vi "AprilTag Desktop.vi"() -> ()   [LabVIEW 2025]
uses:
  <vilib>/Serenial/G Augmented-Reality Toolkit/g_ar_toolkit.feature_detection/Apriltag Detector/Detector Settings.ctl
  <vilib>/Serenial/G Augmented-Reality Toolkit/g_ar_toolkit.capture/Stream/Stream.lvclass/Stream.ctl
  <vilib>/Serenial/G Augmented-Reality Toolkit/g_ar_toolkit.image/New Image (ARGB Preallocated).vi
  <vilib>/Serenial/G Augmented-Reality Toolkit/g_ar_toolkit.image/New Image (Greyscale Preallocated).vi
  <vilib>/Serenial/G Augmented-Reality Toolkit/g_ar_toolkit.capture/Stream/Next Capture (ARGB).vi
  <vilib>/Serenial/G Augmented-Reality Toolkit/g_ar_toolkit.image/Draw Image to Picture (ARGB).vi
  <vilib>/Serenial/G Augmented-Reality Toolkit/g_ar_toolkit.image/ARGB Colour to U32 Pixel Value.vi
  <vilib>/Serenial/G Augmented-Reality Toolkit/g_ar_toolkit.common/NI-Linux-RT Shared Library Path (Core).vi
  <vilib>/Serenial/G Augmented-Reality Toolkit/g_ar_toolkit.image/ARGBExtractChannel.vi
  <vilib>/Serenial/G Augmented-Reality Toolkit/g_ar_toolkit.common/NI-Linux-RT Shared Library Path.vi
  <vilib>/Utility/error.llb/Error Cluster From Error Code.vi
  <vilib>/Serenial/G Augmented-Reality Toolkit/g_ar_toolkit.capture/Stream/Stream.lvclass
  <vilib>/Serenial/G Augmented-Reality Toolkit/g_ar_toolkit.capture/g_ar_toolkit.capture.lvlib
  <vilib>/Serenial/G Augmented-Reality Toolkit/g_ar_toolkit.image/g_ar_toolkit.image.lvlib
  <vilib>/ptbypt/NI_PtbyPt.lvlib
  <vilib>/Serenial/G Augmented-Reality Toolkit/g_ar_toolkit.feature_detection/Apriltag Detector/AprilTag Detector.lvclass
panel:
  out "error out 3":errorcluster
  out "data out":string="2026-03-01 17:38:57"
  out "created path":path=path "/home/wdya/Pictures/Logging/2026-03-01 17:36:43"
  in  "Logging":bool
  out "sorted array":T1(array[cluster])=[{"Particle Report"={"Area"=13859.0, "Number of Holes"=0.0, "Bounding Rect"={"Left"=334.0, "Top"=288.0, "Right"=498.0, "Bottom"=400.0}, "Center of Mass"={"X"=419.3708781297352, "Y"=343.56735695216105}, "Orientation"=170.0255069873374, "Dimensions"={"Width"=164.0, "Height"=112.0}}, "angle"=-138.375, "Distance"=1.235958475021079}, {"Particle Report"={"Area"=8065.0, "Number of Holes"=0.0, "Bounding Rect"={"Left"=1780.0, "Top"=228.0, "Right"=1899.0, "Bottom"=324.0}, "Center of Mass"={"X"=1835.3011779293242, "Y"=272.58115313081214}, "Orientation"=15.20762593083473, "Dimensions"={"Width"=119.0, "Height"=96.0}}, "angle"=39.5625, "Distance"=1.7892920079045385}, {"Particle Report"={"Area"=6502.0, "Number of Holes"=0.0, "Bounding Rect"={"Left"=150.0, "Top"=158.0, "Right"=294.0, "Bottom"=226.0}, "Center of Mass"={"X"=223.40110735158413, "Y"=191.71701015072284}, "Orientation"=172.47240632857867, "Dimensions"={"Width"=144.0, "Height"=68.0}}, "angle"=-162.625, "Distance"=3.1397972320986356}, {"Particle Report"={"Area"=4863.0, "Number of Holes"=0.0, "Bounding Rect"={"Left"=1897.0, "Top"=130.0, "Right"=2023.0, "Bottom"=193.0}, "Center of Mass"={"X"=1956.7361710878058, "Y"=160.65165535677565}, "Orientation"=169.97947489357827, "Dimensions"={"Width"=126.0, "Height"=63.0}}, "angle"=54.625, "Distance"=3.9539909165395755}, {"Particle Report"={"Area"=4522.0, "Number of Holes"=0.0, "Bounding Rect"={"Left"=306.0, "Top"=186.0, "Right"=391.0, "Bottom"=254.0}, "Center of Mass"={"X"=349.0249889429456, "Y"=220.57430340557275}, "Orientation"=175.83587720914608, "Dimensions"={"Width"=85.0, "Height"=68.0}}, "angle"=-146.8125, "Distance"=2.634033890801481}, {"Particle Report"={"Area"=4163.0, "Number of Holes"=0.0, "Bounding Rect"={"Left"=698.0, "Top"=197.0, "Right"=773.0, "Bottom"=270.0}, "Center of Mass"={"X"=735.1179437905357, "Y"=234.18928657218353}, "Orientation"=161.19402599374737, "Dimensions"={"Width"=75.0, "Height"=73.0}}, "angle"=-98.4375, "Distance"=2.397550303556918}, {"Particle Report"={"Area"=3194.0, "Number of Holes"=0.0, "Bounding Rect"={"Left"=1112.0, "Top"=153.0, "Right"=1183.0, "Bottom"=210.0}, "Center of Mass"={"X"=1147.2542266750156, "Y"=181.9909204758923}, "Orientation"=172.9752781561151, "Dimensions"={"Width"=71.0, "Height"=57.0}}, "angle"=-46.9375, "Distance"=3.4981802611246366}, {"Particle Report"={"Area"=2560.0, "Number of Holes"=0.0, "Bounding Rect"={"Left"=1243.0, "Top"=142.0, "Right"=1308.0, "Bottom"=192.0}, "Center of Mass"={"X"=1275.22734375, "Y"=167.34140625}, "Orientation"=178.73331347563146, "Dimensions"={"Width"=65.0, "Height"=50.0}}, "angle"=-30.9375, "Distance"=3.9836910640860386}, {"Particle Report"={"Area"=1543.0, "Number of Holes"=0.0, "Bounding Rect"={"Left"=1321.0, "Top"=117.0, "Right"=1370.0, "Bottom"=156.0}, "Center of Mass"={"X"=1345.0738820479585, "Y"=136.6947504860661}, "Orientation"=174.47565876180477, "Dimensions"={"Width"=49.0, "Height"=39.0}}, "angle"=-22.1875, "Distance"=5.3519881407692065}, {"Particle Report"={"Area"=5191.0, "Number of Holes"=0.0, "Bounding Rect"={"Left"=1230.0, "Top"=32.0, "Right"=1460.0, "Bottom"=84.0}, "Center of Mass"={"X"=1330.0730109805434, "Y"=58.25332305914082}, "Orientation"=178.73286326372457, "Dimensions"={"Width"=230.0, "Height"=52.0}}, "angle"=-22.25, "Distance"=12.765326788205794}]
  out "loop time (s) 2":dbl=0.218
  in  "Detector Settings":T2={"Refine Edges (Default: True)"=TRUE, "Threads (Default: 1)"=3, "Decimate (Default: 1)"=2.0, "Blur (Default: 0)"=0.0, "Bits (Default: 2)"=2} {"Threads (Default: 1)" min=1}
  out "2D Picture 2":picture
  out "Waveform Chart":dbl(graph)=0.089
  out "detect":dbl=0.04548390699983429
  out "gray":dbl
  in  "dbg index":i32=-2
  in  "slices":i32=2
  in  "Display":bool
  out "2D Picture":picture
  out "Acquire":dbl=0.08587937099991905
  out "Timed Out?":bool
  out "Filtered x":dbl=77.7800196035477 format="%0.2f"
  out "median of 5":dbl=78.0 format="%0.2f"
  in  "Stop":bool
  out "error out 2":errorcluster
  in  "camera index":i32
  in  "Circle Config":T3={"Sorting Mode"=enum."Furthest Away", "How Many Circles?"=3.0}
  out "Tag & Angle":cluster{"tag ID":i32, "angle":dbl}[](array[cluster])=[{"tag ID"=7, "angle"=-41.30036333562276}, {"tag ID"=9, "angle"=5.5491101303770165}, {"tag ID"=10, "angle"=8.973745640321852}]
  out "Array 2":cluster{"tag ID":i32, "tag ID":i32, dbl}[](array[cluster])=[{"tag ID"=7, "tag ID"=9, 46.84947346599978}, {"tag ID"=7, "tag ID"=10, 50.274108975944614}, {"tag ID"=9, "tag ID"=10, 3.424635509944835}]
  in  "Angle Mode":enum16{"Barrel View", "360 View"}(ring)=enum."360 View"
  in  "Split Image Info":T4={"height"=1024, "width"=1920, "deg/pix"=0.178}
  in  "tag info not from game manual":dbl[][](array[numeric])=[[6.0, 13.21, 0.0, 2.0, 0.0], [7.0, 26.4, 7.0, 1.0, 270.0], [11.0, 0.0, 7.0, 1.0, 90.0], [-1.0, 24.2667, 2.7924999999999995, 4.875, 306.0], [-1.0, 13.21, 0.0, 4.0, 0.0], [10.0, 2.15003, 2.7925, 4.875, 54.0], [-1.0, 13.21, 0.0, 5.875, 0.0], [17.0, 7.21, 0.0, 2.0, 0.0], [-1.0, 7.21, 0.0, 4.0, 0.0], [-1.0, 7.21, 0.0, 5.875, 0.0]]
  in  "IMU value":dbl=32.15 format="%#_13g"
  in  "Circles":bool
  in  "Chords":bool
  in  "Lines":bool
  in  "IMU offset":dbl
  out "Tags":T5(array[cluster])=[{"tag info"={"tag ID"=7, "Center"={"X"=1109.597093315018, "Y"=662.2761466988038}, "Homography Matrix"=[], "dec margin"=98.43096160888672, "Hamming Dist"=0, "Corner Points"=[{"X"=1099.6268310546875, "Y"=672.8292846679686}, {"X"=1119.9018554687502, "Y"=672.0942993164062}, {"X"=1119.3701171875, "Y"=651.9317779541016}, {"X"=1099.2615966796875, "Y"=652.4287109375}], "Tag Family"=""}, {"angle"=-41.30036333562276, "field locations (ft)"={"X"=24.404, "Y"=39.169}}}, {"tag info"={"tag ID"=9, "Center"={"X"=1484.3928810430161, "Y"=638.7891766343314}, "Homography Matrix"=[], "dec margin"=57.157508850097656, "Hamming Dist"=1, "Corner Points"=[{"X"=1477.2242431640623, "Y"=646.967559814453}, {"X"=1490.9765625, "Y"=648.1733093261719}, {"X"=1491.1896972656252, "Y"=631.0349884033203}, {"X"=1477.414306640625, "Y"=628.8421783447266}], "Tag Family"=""}, {"angle"=5.5491101303770165, "field locations (ft)"={"X"=14.448, "Y"=41.028}}}, {"tag info"={"tag ID"=10, "Center"={"X"=1511.7899651225748, "Y"=642.6690792487474}, "Homography Matrix"=[], "dec margin"=56.893287658691406, "Hamming Dist"=0, "Corner Points"=[{"X"=1505.5390625000002, "Y"=650.0198974609375}, {"X"=1517.7366943359377, "Y"=651.9248352050781}, {"X"=1518.1419677734375, "Y"=635.1993713378906}, {"X"=1505.7580566406248, "Y"=633.2807464599609}], "Tag Family"=""}, {"angle"=8.973745640321852, "field locations (ft)"={"X"=13.282, "Y"=41.028}}}]
  out "loop time (s)":dbl=0.089
  out "Field":cluster{cluster{"X":dbl, "Y":dbl}[]}[](graph)
  # "Angles between\ntarget and camera"
  # "order:\n6\n7\n11\n18\n20\n10\n22\n17\n19\n21"
  # "Offset between\ntarget and camera"
  # "Better way to pick camera matrix\ncheck other cams and simplify scaling"
  # "dec1 three threads 60 to 70 ms for april"
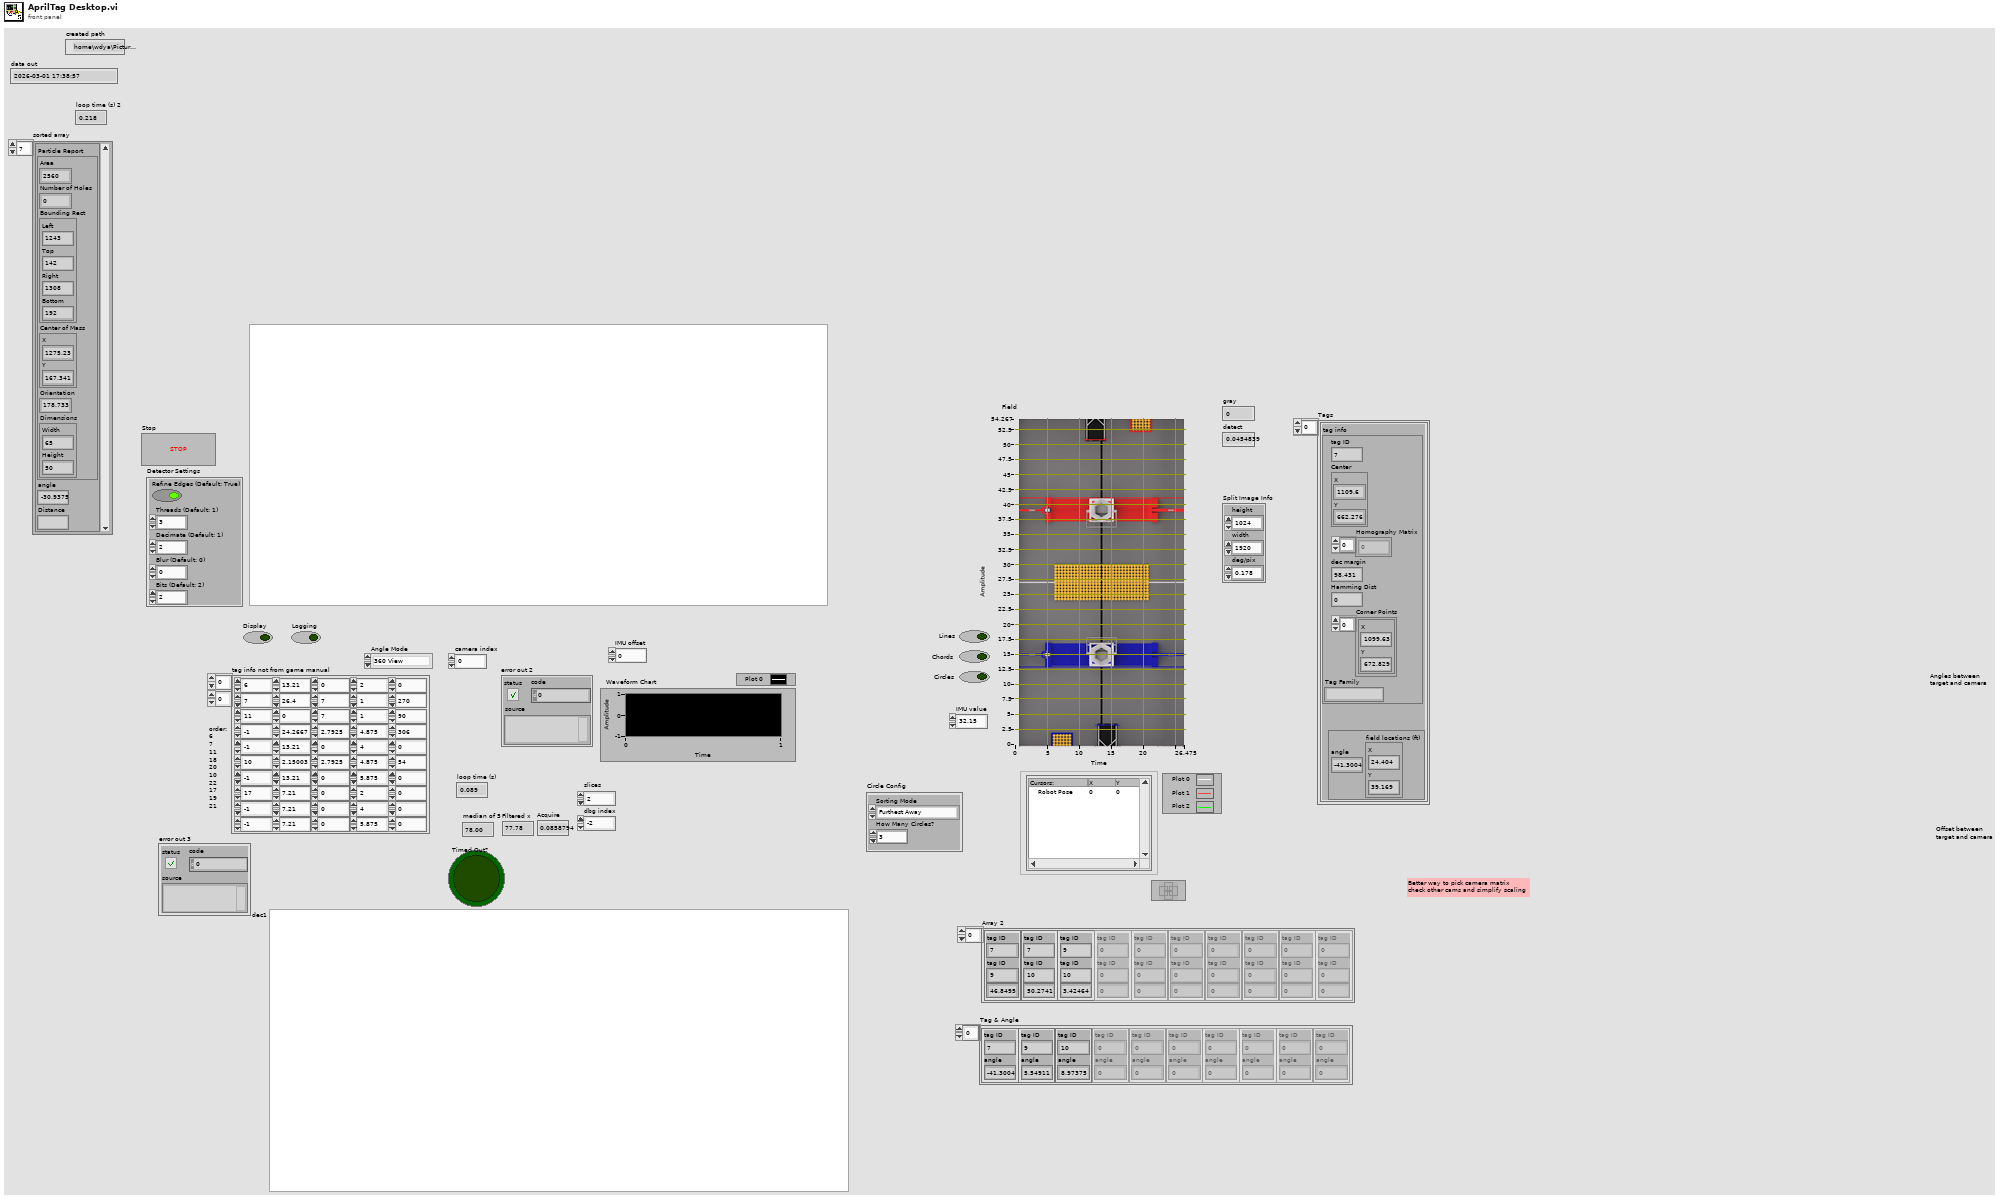
[diagram p1: front panel]
types:
  T1 = cluster{"Particle Report":cluster{"Area":dbl, "Number of Holes":dbl, "Bounding Rect":cluster{"Left":dbl, "Top":dbl, "Right":dbl, "Bottom":dbl}, "Center of Mass":cluster{"X":dbl, "Y":dbl}, "Orientation":dbl, "Dimensions":cluster{"Width":dbl, "Height":dbl}}, "angle":dbl, "Distance":ext}[]
  T2 = typedef "g_ar_toolkit.feature_detection.lvlib/AprilTag Detector.lvclass/Detector Settings.ctl" = cluster{"Refine Edges (Default: True)":bool, "Threads (Default: 1)":u8, "Decimate (Default: 1)":sgl, "Blur (Default: 0)":sgl, "Bits (Default: 2)":u8}
  T3 = cluster{"Sorting Mode":enum16{"Furthest Away", "Largest Radius"}, "How Many Circles?":dbl}
  T4 = cluster{"height":i32, "width":i32, "deg/pix":dbl}
  T5 = cluster{"tag info":cluster{"tag ID":i32, "Center":cluster{"X":dbl, "Y":dbl}, "Homography Matrix":dbl[], "dec margin":dbl, "Hamming Dist":i32, "Corner Points":cluster{"X":dbl, "Y":dbl}[], "Tag Family":string}, cluster{"angle":dbl, "field locations (ft)":cluster{"X":dbl, "Y":dbl}}}[]
  T6 = typedef "Image Type" = u32
  T7 = cluster{"Name":string, "Color":u32, "Style":i32, "Point Style":i32, "Name Visible":bool, "Allow Drag":bool, "Cursor Mode":u32, "Plot":i32, "Index":i32, "Position":cluster{"X":dbl, "Y":dbl}, "X Scale":u32, "Y Scale":u32, "Watch Plots":i32[], "Watch All Plots":bool, "Plot Area":i32, "Label Offset":cluster{"X":i32, "Y":i32}}
  T8 = cluster{i32, "Position":cluster{"X":dbl, "Y":dbl}}[]
  T9 = typedef "g_ar_toolkit.capture.lvlib/Stream.lvclass/Stream Specification.ctl" = cluster{"Size":T10, "FPS":T11}
  T10 = typedef "g_ar_toolkit.common.lvlib/Image Size (Integer).ctl" = cluster{"Width":u16, "Height":u16}
  T11 = typedef "g_ar_toolkit.capture.lvlib/Stream.lvclass/Frames per Second.ctl" = cluster{"Numerator":u32, "Denominator":u32}
  T12 = cluster{"ID":string, "Name":string, "Stream Specifications":T9[]}[]
  T13 = cluster{"ID":string, "Name":string, "Stream Specifications":T9[]}
  T14 = typedef "g_ar_toolkit.image.lvlib/ARGB Image.ctl" = refnum<data-value>
  T15 = typedef "IMAQ Image.ctl" = refnum<image>
  T16 = typedef "g_ar_toolkit.image.lvlib/Greyscale Image.ctl" = refnum<data-value>
  T17 = enum16{"open", "replace", "create", "open or create", "replace or create", "replace or create with confirmation"}
  T18 = typedef "g_ar_toolkit.feature_detection.lvlib/AprilTag Detector.lvclass/Detection.ctl" = cluster{"ID":i32, "Hamming":i32, "Decision Margin":sgl, "Centre":T19, "Corners":T20}
  T19 = typedef "g_ar_toolkit.common.lvlib/Image Point (Float).ctl" = cluster{"x":dbl, "y":dbl}
  T20 = typedef "g_ar_toolkit.common.lvlib/Quad Corners.ctl" = cluster{"Bottom Left":T19, "Bottom Right":T19, "Top Right":T19, "Top Left":T19}
  T21 = cluster{"tag info":cluster{"tag ID":i32, "Center":cluster{"X":dbl, "Y":dbl}, "Homography Matrix":dbl[], "dec margin":dbl, "Hamming Dist":i32, "Corner Points":cluster{"X":dbl, "Y":dbl}[], "Tag Family":string}, "Ange + Field Pos":cluster{"angle":dbl, "field locations (ft)":cluster{"X":dbl, "Y":dbl}}}[]
  T22 = cluster{"Tag 1":cluster{"tag info":cluster{"tag ID":i32, "Center":cluster{"X":dbl, "Y":dbl}, "Homography Matrix":dbl[], "dec margin":dbl, "Hamming Dist":i32, "Corner Points":cluster{"X":dbl, "Y":dbl}[], "Tag Family":string}, cluster{"angle":dbl, "field locations (ft)":cluster{"X":dbl, "Y":dbl}}}, "Tag 2":cluster{"tag info":cluster{"tag ID":i32, "Center":cluster{"X":dbl, "Y":dbl}, "Homography Matrix":dbl[], "dec margin":dbl, "Hamming Dist":i32, "Corner Points":cluster{"X":dbl, "Y":dbl}[], "Tag Family":string}, cluster{"angle":dbl, "field locations (ft)":cluster{"X":dbl, "Y":dbl}}}}[]
  T23 = cluster{"Tag 1":cluster{"tag info":cluster{"tag ID":i32, "Center":cluster{"X":dbl, "Y":dbl}, "Homography Matrix":dbl[], "dec margin":dbl, "Hamming Dist":i32, "Corner Points":cluster{"X":dbl, "Y":dbl}[], "Tag Family":string}, "Angle + Field Pos":cluster{"angle":dbl, "field locations (ft)":cluster{"X":dbl, "Y":dbl}}}, "Tag 2":cluster{"tag info":cluster{"tag ID":i32, "Center":cluster{"X":dbl, "Y":dbl}, "Homography Matrix":dbl[], "dec margin":dbl, "Hamming Dist":i32, "Corner Points":cluster{"X":dbl, "Y":dbl}[], "Tag Family":string}, "Angle + Field Pos":cluster{"angle":dbl, "field locations (ft)":cluster{"X":dbl, "Y":dbl}}}}[]
  T24 = cluster{"tag info":cluster{"tag ID":i32, "Center":cluster{"X":dbl, "Y":dbl}, "Homography Matrix":dbl[], "dec margin":dbl, "Hamming Dist":i32, "Corner Points":cluster{"X":dbl, "Y":dbl}[], "Tag Family":string}, "Angle + Field Pos":cluster{"angle":dbl, "field locations (ft)":cluster{"X":dbl, "Y":dbl}}}
  T25 = cluster{"angle":dbl, "field locations (ft)":cluster{"X":dbl, "Y":dbl}}
  T26 = cluster{"Angle + Field Pos":cluster{"angle":dbl, "field locations (ft)":cluster{"X":dbl, "Y":dbl}}, "Angle + Field Pos":cluster{"angle":dbl, "field locations (ft)":cluster{"X":dbl, "Y":dbl}}}
  T27 = cluster{"center":cluster{"X":sgl, "Y":sgl}, "radius":sgl}
  T28 = cluster{"output circle info":cluster{"center":cluster{"X":sgl, "Y":sgl}, "radius":sgl}, cluster{"Points":cluster{dbl, dbl}[]}}
  T29 = cluster{"center":cluster{"X":sgl, "Y":sgl}, "radius":sgl}[]
  T30 = cluster{"Name":string, "Color":u32, "Style":i32, "Point Style":i32, "Name Visible":bool, "Allow Drag":bool, "Cursor Mode":u32, "Plot":i32, "Index":i32, "Position":cluster{"X":dbl, "Y":dbl}, "X Scale":u32, "Y Scale":u32, "Watch Plots":i32[], "Watch All Plots":bool, "Plot Area":i32, "Label Offset":cluster{"X":i32, "Y":i32}}[]
  T31 = cluster{"Detections":T18[], "Robot Pose":cluster{dbl, dbl}, "sorted array":cluster{"Particle Report":cluster{"Area":dbl, "Number of Holes":dbl, "Bounding Rect":cluster{"Left":dbl, "Top":dbl, "Right":dbl, "Bottom":dbl}, "Center of Mass":cluster{"X":dbl, "Y":dbl}, "Orientation":dbl, "Dimensions":cluster{"Width":dbl, "Height":dbl}}, "angle":dbl, "Distance":ext}[]}
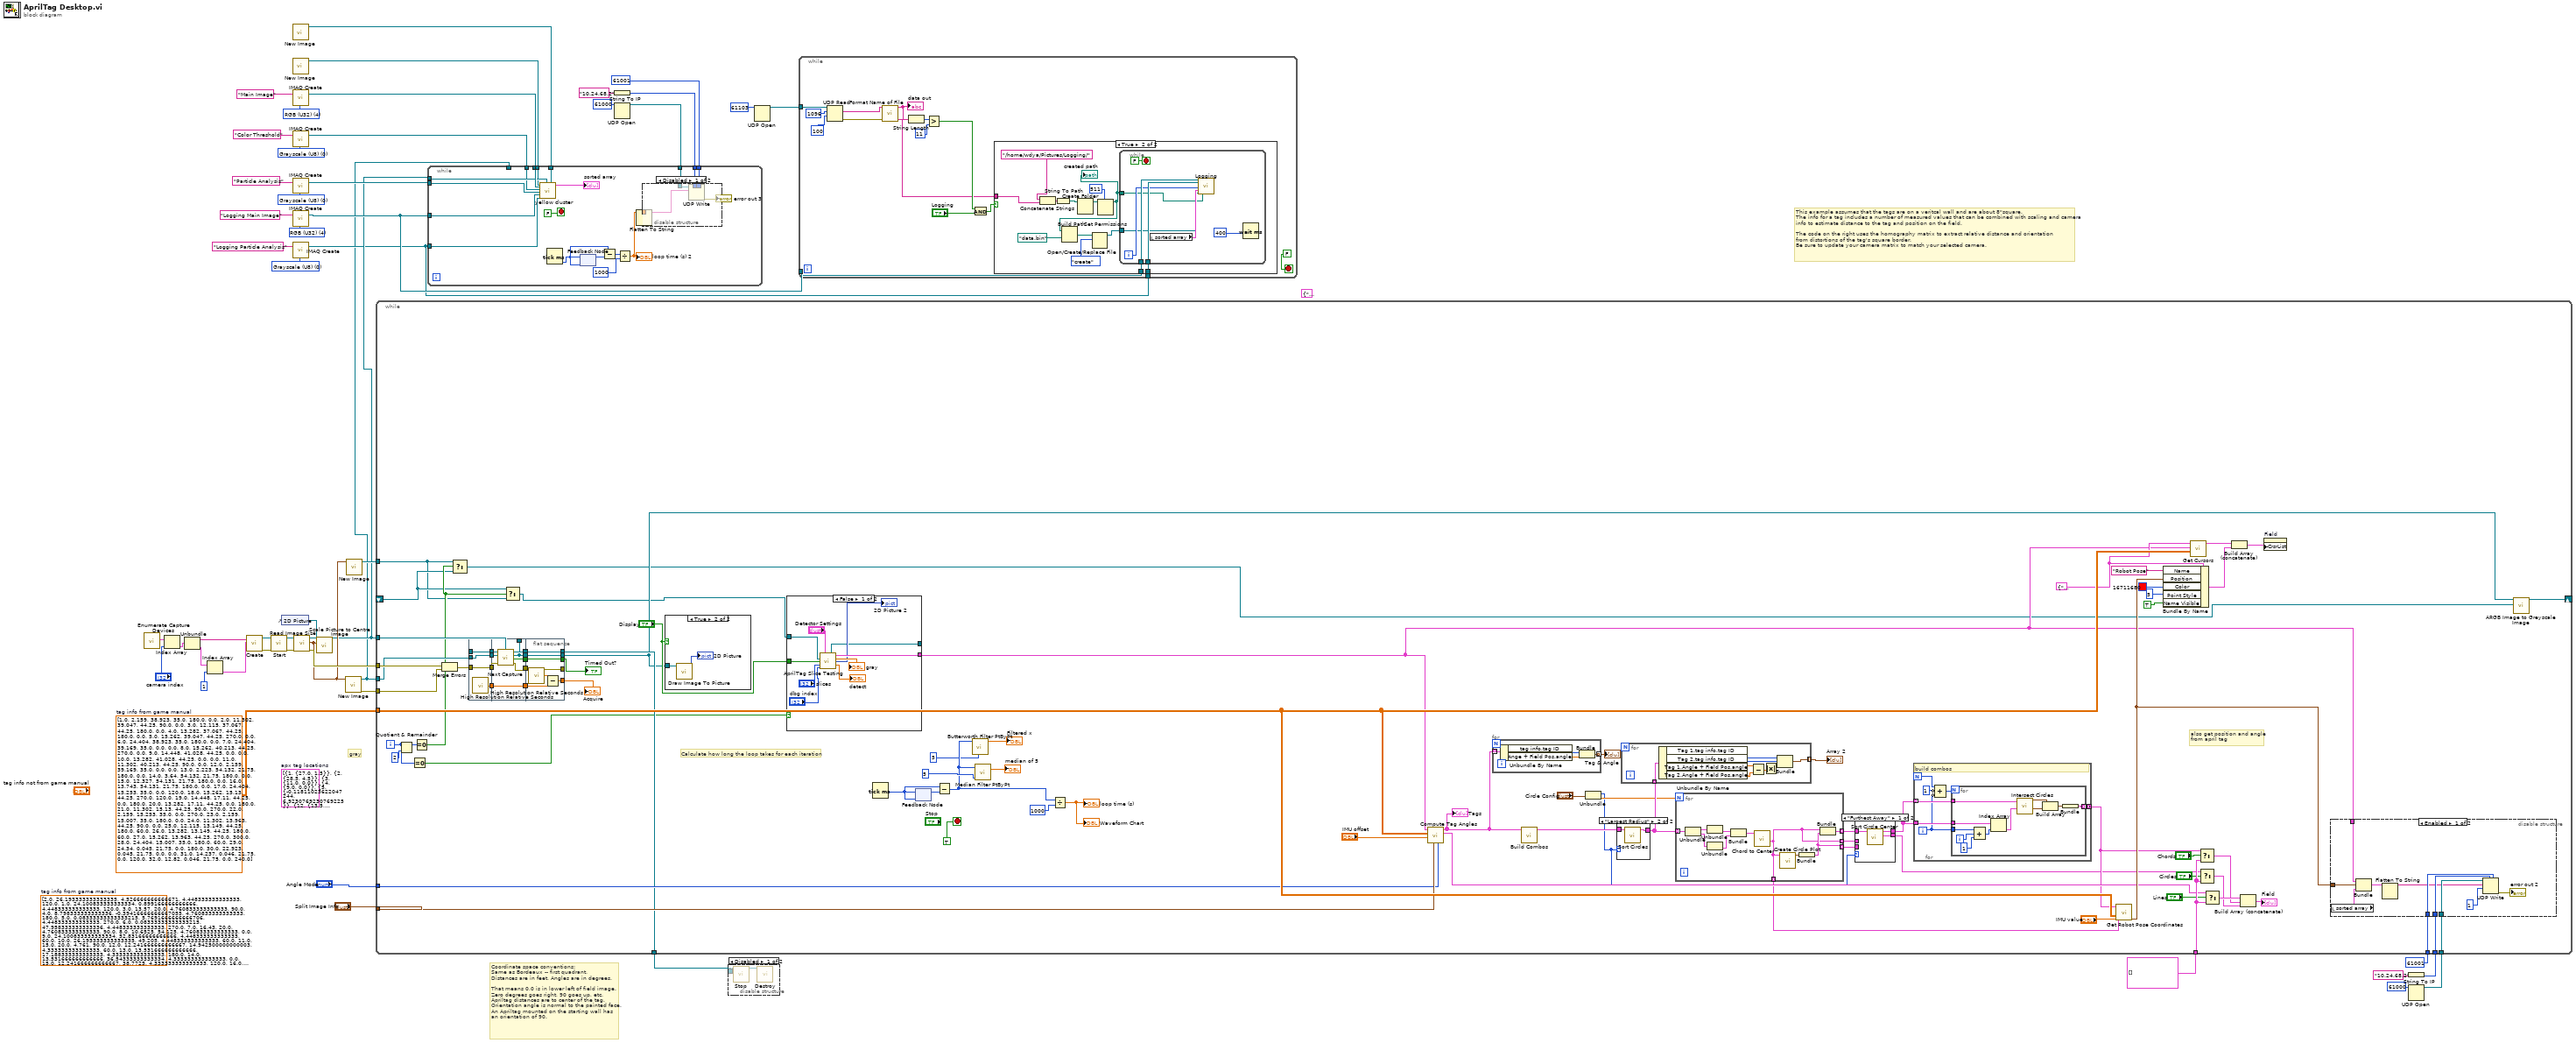
[diagram p0: block diagram]
diagram:
  w13 = T6 0 items=["Grayscale (U8)", "Grayscale (I16)", "Grayscale (SGL)", "Complex (CSG)", "RGB (U32)", "HSL (U32)", "RGB (U64)", "Grayscale (U16)"] ("Image Type")
  w15 = T6 4 items=["Grayscale (U8)", "Grayscale (I16)", "Grayscale (SGL)", "Complex (CSG)", "RGB (U32)", "HSL (U32)", "RGB (U64)", "Grayscale (U16)"] ("Image Type")
  w21 = T6 4 items=["Grayscale (U8)", "Grayscale (I16)", "Grayscale (SGL)", "Complex (CSG)", "RGB (U32)", "HSL (U32)", "RGB (U64)", "Grayscale (U16)"] ("Image Type")
  w23 = T6 0 items=["Grayscale (U8)", "Grayscale (I16)", "Grayscale (SGL)", "Complex (CSG)", "RGB (U32)", "HSL (U32)", "RGB (U64)", "Grayscale (U16)"] ("Image Type")
  w25 = T6 0 items=["Grayscale (U8)", "Grayscale (I16)", "Grayscale (SGL)", "Complex (CSG)", "RGB (U32)", "HSL (U32)", "RGB (U64)", "Grayscale (U16)"] ("Image Type")
  (unwired) T7 {"Name"="", "Color"=61192, "Style"=4, "Point Style"=6, "Name Visible"=TRUE, "Allow Drag"=TRUE, "Cursor Mode"=0, "Plot"=0, "Index"=0, "Position"={"X"=0.0, "Y"=0.0}, "X Scale"=0, "Y Scale"=0, "Watch Plots"=[], "Watch All Plots"=FALSE, "Plot Area"=0, "Label Offset"={"X"=1, "Y"=1}}
  (unwired) dbl[][] [[2.0, 26.193333333333335, 4.526666666666671, 4.448333333333333, 120.0], [1.0, 24.100833333333334, 0.899166666666666, 4.448333333333333, 120.0], [3.0, 13.57, 20.0, 4.760833333333333, 90.0], [4.0, 8.798333333333336, -0.39416666666667055, 4.760833333333333, 180.0], [5.0, 0.08333333333333215, 5.7691666666666706, 4.448333333333333, 270.0], [6.0, 0.08333333333333215, 47.958333333333336, 4.448333333333333, 270.0], [7.0, 16.43, 20.0, 4.760833333333333, 90.0], [8.0, 10.6525, 54.125, 4.760833333333333, 0.0], [9.0, 24.100833333333334, 52.83166666666666, 4.448333333333333, 60.0], [10.0, 26.193333333333335, 49.205, 4.448333333333333, 60.0], [11.0, 15.0, 20.0, 4.761, 90.0], [12.0, 12.241666666666667, 14.942500000000003, 4.333333333333333, 60.0], [13.0, 13.531666666666666, 17.188333333333333, 4.333333333333333, 180.0], [14.0, 13.531666666666666, 36.54333333333334, 4.333333333333333, 0.0], [15.0, 12.241666666666667, 38.7725, 4.333333333333333, 120.0], [16.0, 14.8175, 38.7725, 4.333333333333333, 240.0]]  # tag info from game manual
  w39 = dbl[][] [[1.0, 2.159, 38.923, 35.0, 180.0, 0.0], [2.0, 11.302, 39.047, 44.25, 90.0, 0.0], [3.0, 12.115, 37.067, 44.25, 180.0, 0.0], [4.0, 13.282, 37.067, 44.25, 180.0, 0.0], [5.0, 15.262, 39.047, 44.25, 270.0, 0.0], [6.0, 24.404, 38.923, 35.0, 180.0, 0.0], [7.0, 24.404, 39.169, 35.0, 0.0, 0.0], [8.0, 15.262, 40.213, 44.25, 270.0, 0.0], [9.0, 14.448, 41.028, 44.25, 0.0, 0.0], [10.0, 13.282, 41.028, 44.25, 0.0, 0.0], [11.0, 11.302, 40.213, 44.25, 90.0, 0.0], [12.0, 2.159, 39.169, 35.0, 0.0, 0.0], [13.0, 2.223, 54.132, 21.75, 180.0, 0.0], [14.0, 3.64, 54.132, 21.75, 180.0, 0.0], [15.0, 12.327, 54.131, 21.75, 180.0, 0.0], [16.0, 13.743, 54.131, 21.75, 180.0, 0.0], [17.0, 24.404, 15.253, 35.0, 0.0, 120.0], [18.0, 15.262, 15.13, 44.25, 270.0, 120.0], [19.0, 14.448, 17.11, 44.25, 0.0, 180.0], [20.0, 13.282, 17.11, 44.25, 0.0, 180.0], [21.0, 11.302, 15.13, 44.25, 90.0, 270.0], [22.0, 2.159, 15.253, 35.0, 0.0, 270.0], [23.0, 2.159, 15.007, 35.0, 180.0, 0.0], [24.0, 11.302, 13.963, 44.25, 90.0, 0.0], [25.0, 12.115, 13.149, 44.25, 180.0, 60.0], [26.0, 13.282, 13.149, 44.25, 180.0, 60.0], [27.0, 15.262, 13.963, 44.25, 270.0, 300.0], [28.0, 24.404, 15.007, 35.0, 180.0, 60.0], [29.0, 24.34, 0.045, 21.75, 0.0, 180.0], [30.0, 22.923, 0.045, 21.75, 0.0, 0.0], [31.0, 14.237, 0.046, 21.75, 0.0, 120.0], [32.0, 12.82, 0.046, 21.75, 0.0, 240.0]]  # tag info from game manual
  (unwired) T8 [{1, "Position"={"X"=27.0, "Y"=1.5}}, {2, "Position"={"X"=28.5, "Y"=4.5}}, {3, "Position"={"X"=11.0, "Y"=0.0}}, {4, "Position"={"X"=9.0, "Y"=0.0}}, {5, "Position"={"X"=-0.11811023622047244, "Y"=6.9230769230769225}}, {12, "Position"={"X"=13.5, "Y"=17.0}}]  # apx tag locations
  # "gray"
  # "Coordinate space conventions:\nSame as Bordeaux -- first quadrant.\nDistances are in feet. Angles are in degrees.\n\nThat means 0,0 is in lower left of field image.\nZero degrees goes right, 90 goes up, etc.\nApriltag distances are to center of the tag.\nOrientation angle is normal to the painted face.\nAn Apriltag mounted on the starting wall has\nan orientation of 90."
  # "This example assumes that the tags are on a veritcal wall and are about 8\"square. \nThe info for a tag includes a number of measured values that can be combined with scaling and camera\ninfo to estimate distance to the tag and position on the field. \n\nThe code on the right uses the homography matrix to extract relative distance and orientation\nfrom distortions of the tag's square border.\nBe sure to update your camera matrix to match your selected camera."
  n1 = call <vilib>:"Enumerate Capture Devices.vi"() -> ("Devices"=w46:T12)  [unwired: 10 in, 1 out]
  n2 = Index Array(array=w46, index="camera index") -> (element=w47:T13)
  n3 = Unbundle(w47) -> ("ID"=w48:string, "Stream Specifications"=w49:T9[])  [unwired: 1 out]
  n4 = Index Array(array=w49, index=1) -> (element=w36:T9)
  n5 = call <vilib>:"Create.vi"("Desired Stream Specification"=w36, "Device ID"=w48) -> ("error out"=w44:errorcluster, "Stream"=w43:refnum<class "Stream.lvclass">)  [unwired: 8 in]
  n6 = call <vilib>:"Start.vi"("error in (no error)"=w44, "Stream in"=w43) -> ("error out"=w45:errorcluster, "Stream"=w42:refnum<class "Stream.lvclass">)  [unwired: 8 in]
  n7 = control-ref of="2D Picture"() -> (w29:refnum<vi>)
  n8 = call-poly <vilib>:"New Image.vi"() -> ("ARGB Image"=w18:T14)  [unwired: 10 in, 1 out]
  n9 = call-poly <vilib>:"New Image.vi"() -> ("ARGB Image"=w19:T14)  [unwired: 10 in, 1 out]
  n10 = call "IMAQ Create"("Image Name"="Main Image", "Image Type"=w21) -> ("New Image"=w17:T15)  [unwired: 3 in, 1 out]
  n11 = call "IMAQ Create"("Image Name"="Color Threshold", "Image Type"=w25) -> ("New Image"=w20:T15)  [unwired: 3 in, 1 out]
  n12 = call "IMAQ Create"("Image Name"="Particle Analysis", "Image Type"=w23) -> ("New Image"=w16:T15)  [unwired: 3 in, 1 out]
  n13 = call "IMAQ Create"("Image Name"="Logging Main Image", "Image Type"=w15) -> ("New Image"=w11:T15)  [unwired: 3 in, 1 out]
  n14 = call "IMAQ Create"("Image Name"="Logging Particle Analysis", "Image Type"=w13) -> ("New Image"=w7:T15)  [unwired: 3 in, 1 out]
  n15 = call <vilib>:"Read Image Size.vi"("error in (no error)"=w45, "Stream in"=w42) -> ("error out"=w37:errorcluster, "Image Size"=w28:T10, "Stream"=w8:refnum<class "Stream.lvclass">)  [unwired: 7 in]
  n16 = call <vilib>:"Scale Picture to Centre Image.vi"("Image Size"=w28, "Picture in"=w29) -> ()  [unwired: 7 in, 3 out]
  n17 = call-poly <vilib>:"New Image.vi"("Preallocated Image Size (Default: 0,0)"=w28) -> ("error out"=w38:errorcluster, "ARGB Image"=w6:T14)  [unwired: 9 in]
  n18 = call-poly <vilib>:"New Image.vi"("Preallocated Image Size (Default 0,0)"=w28) -> ("Greyscale Image"=w27:T16)  [unwired: 9 in, 1 out]
  n19 = String To IP(1:"10.24.68.2" ("name")) -> (0:w2:u32)
  n20 = UDP Open(11:u16 61000 ("port")) -> (port=w1:refnum<k16>)  [unwired: 4 in, 2 out]
  n21 = while {
    tunnel: w16 -> [w59]
    tunnel: w20 -> [w60]
    tunnel: w17 -> [w70]
    tunnel: w19 -> [w61]
    tunnel: w18 -> [w69]
    tunnel: w8 -> [w62]
    tunnel: w11 -> [w58]
    tunnel: w7 -> [w57]
    tunnel: w6 -> [_]
    tunnel: u16 61001 -> [w56]
    tunnel: w2 -> [w54]
    tunnel: w1 -> [w53]
    stop <- FALSE stop-if-true
    n22 = call "yellow cluster.vi"("Cropped Image"=w61, "Main Image"=w70, "Color Threshold"=w60, "Particle Analysis"=w59, "Logging Main Image"=w58, "Logging Particle Analysis"=w57, "Stream"=w62, "Image"=w69) -> ("sorted array"=→"sorted array":T1)  [unwired: 11 in]
    n23 = Tick Count (ms)() -> (millisecond timer value=w66:u32)
    n24 = feedback #1(w66) -> (w67:u32)
    n25 = feedback-in #1(w66) -> ()
    n26 = Subtract(x=w66, y=w67) -> (x-y=w65:u32)
    n27 = Divide(x=w65, y=1000) -> (x/y=w55:dbl)
    "loop time (s) 2" <- w55
    n28 = disable-structure shown="Disabled" {
      disable-tunnel: w56 -> [w75 _]
      disable-tunnel: w55 -> [w73 _]
      disable-tunnel: w54 -> [w72 _]
      disable-tunnel: w53 -> [w71 _]
      frame Disabled {
        n29 = Flatten To String(anything=w73) -> (data string=w74:string)  [unwired: 3 in, 2 out]
        n30 = UDP Write(address=w72, port or service name=w75, connection ID=w71, data in=w74) -> (error out=→"error out 3":errorcluster)  [unwired: 2 in, 1 out]
      }
      frame Enabled {
      }
    }
  }
  n31 = UDP Open(11:u16 61103 ("port")) -> (port=w9:refnum<k16>)  [unwired: 4 in, 2 out]
  n32 = while {
    tunnel: w11 -> [w91]
    tunnel: w7 -> [w90]
    tunnel: w9 -> [w87]
    stop <- FALSE stop-if-true
    n33 = UDP Read(connection ID=w87, max size (548)=1096, timeout ms (25000)=100) -> (data out=w78:string, error out=w83:errorcluster)  [unwired: 1 in, 3 out]
    n34 = call "Format Name of File.vi"("error in (no error)"=w83, "data in"=w78) -> ("Name of File"=w77:string, "Time String"=w82:string)  [unwired: 8 in]
    "data out" <- w82
    n35 = String Length(string=w82) -> (length=w81:i32)
    n36 = Greater?(x=w81, y=11) -> (0:w79:bool)
    n37 = And(x=w79, y="Logging") -> (x .and. y?=w85:bool)
    n38 = case shown="True" w85 {
      tunnel: w91 -> [_ w104]
      tunnel: w90 -> [_ w103]
      tunnel: w77 -> [_ w92]
      frame False {
      }
      frame True {
        n39 = Concatenate Strings("/home/wdya/Pictures/Logging/", w92) -> (w97:string)
        n40 = String To Path(string=w97) -> (path=w95:path)
        n41 = Create Folder(path (use dialog)=w95) -> (created path=w94:path)  [unwired: 2 in, 2 out]
        n42 = Set Permissions(7:i16 511 ("permissions"), 11:w94) -> (3:w93:path)  [unwired: 3 in, 1 out]
        "created path" <- w93
        n43 = Build Path(base path=w93, name or relative path=path "data.bin") -> (appended path=w100:path)
        n44 = Open/Create/Replace File(file path (use dialog)=w100, operation (0:open)=T17."create") -> (refnum out=w99:refnum<file>)  [unwired: 4 in, 2 out]
        n45 = while {
          tunnel: w104 -> [w110]
          tunnel: w103 -> [w109]
          tunnel: w93 -> [w106]
          tunnel: w99 -> [w105]
          i -> [w108]
          stop <- FALSE stop-if-true
          n46 = local read "sorted array"() -> (w107:T1)
          n47 = call "Logging.vi"("Main Image"=w110, "Particle Analysis"=w109, "Index"=w108, "sorted array 2"=w107, "refnum out"=w105, "Path"=w106) -> ()  [unwired: 14 in]
          n48 = Wait (ms)(milliseconds to wait=u32 400) -> ()  [unwired: 1 out]
        }
      }
    }
  }
  n49 = String To IP(1:"10.24.68.2" ("name")) -> (0:w32:u32)
  n50 = UDP Open(11:u16 61000 ("port")) -> (port=w31:refnum<k16>)  [unwired: 4 in, 2 out]
  n51 = while {
    tunnel: w39 -> [w189]
    tunnel: cluster{cluster{"X":dbl, "Y":dbl}[]}[] [] ("Vectors") -> [w190]
    tunnel: "Split Image Info" -> [w188]
    tunnel: "Angle Mode" -> [w187]
    tunnel: w8 -> [w186]
    tunnel: w6 -> [w119]
    tunnel: w38 -> [w185]
    tunnel: w37 -> [w184]
    tunnel: u16 61001 -> [w182]
    tunnel: w32 -> [w181]
    tunnel: w31 -> [w180]
    tunnel: [w163] -> w30
    shift-right: [w121] -> _
    shift-left: _ -> [w115]
    tunnel: w27 -> [w114]
    i -> [w124]
    stop <- TRUE stop-if-true
    w162 = T7 {"Name"="", "Color"=61192, "Style"=4, "Point Style"=6, "Name Visible"=TRUE, "Allow Drag"=TRUE, "Cursor Mode"=0, "Plot"=0, "Index"=0, "Position"={"X"=0.0, "Y"=0.0}, "X Scale"=0, "Y Scale"=0, "Watch Plots"=[], "Watch All Plots"=FALSE, "Plot Area"=0, "Label Offset"={"X"=1, "Y"=1}}
    # "also get position and angle\nfrom april tag"
    # "Calculate how long the loop takes for each iteration"
    n52 = Quotient & Remainder(x=w124, y=2) -> (x-y*floor(x/y)=w125:i32)  [unwired: 1 out]
    n53 = Equal To 0?(x=w124) -> (x = 0?=w123:bool)
    n54 = Equal To 0?(x=w125) -> (x = 0?=w117:bool)
    n55 = Merge Errors(w184, w185) -> (w183:errorcluster)
    n56 = Select(t=w114, s=w117, f=w115) -> (s? t:f=w116:T16)
    n57 = flat-sequence {
      tunnel: w183 -> [w256]
      tunnel: w186 -> [w257]
      tunnel: [w257] -> w168
      tunnel: [w256] -> w167
      tunnel: [w255] -> w165
      tunnel: [w254] -> w120
      tunnel: w119 -> [w254]
      tunnel: [w258] -> w172
      tunnel: [w263] -> w171
      tunnel: [w262] -> w170
      tunnel: [w261] -> w169
      tunnel: w168 -> [w265]
      tunnel: w167 -> [w264]
      tunnel: [w260] -> w166
      tunnel: w165 -> [w260]
      tunnel: w120 -> [w259]
      tunnel: [w258] -> _
      tunnel: [w270] -> w173
      tunnel: [w271] -> w163
      tunnel: [w272] -> _
      tunnel: w172 -> [w266]
      tunnel: w171 -> [w272]
      tunnel: w170 -> [w271]
      tunnel: w169 -> [w270]
      tunnel: w166 -> [w269]
      tunnel: [w267] -> w164
      tunnel: [w266] -> w122
      frame #0 {
        n58 = call <vilib>:"High Resolution Relative Seconds.vi"() -> ("relative seconds"=w255:dbl)
      }
      frame #1 {
        n59 = call-poly <vilib>:"Next Capture.vi"("error in (no error)"=w264, "ARGB Destination Image in"=w259, "Stream in"=w265) -> ("error out"=w263:errorcluster, "Timed Out?"=w261:bool, "ARGB Destination Image"=w258:T14, "Stream"=w262:refnum<class "Stream.lvclass">)  [unwired: 5 in]
      }
      frame #2 {
        n60 = call <vilib>:"High Resolution Relative Seconds.vi"() -> ("relative seconds"=w268:dbl)
        n61 = Subtract(x=w268, y=w269) -> (x-y=w267:dbl)
      }
    }
    n62 = Select(t=w115, s=w117, f=w114) -> (s? t:f=w118:T16)
    n63 = case shown="True" "Display" {
      tunnel: w122 -> [_ w204]
      frame False {
      }
      frame True {
        n64 = call-poly <vilib>:"Draw Image To Picture.vi"("ARGB Image Source in"=w204) -> ("Picture"=→"2D Picture":picture)  [unwired: 9 in, 1 out]
      }
    }
    n65 = case shown="False" w123 {
      tunnel: [w203 _] -> w129
      tunnel: "Display" -> [w198 _]
      tunnel: w118 -> [w195 _]
      tunnel: [w194 _] -> _
      frame False {
        n66 = call "AprilTag Slice Testing.vi"("Detector Settings"="Detector Settings", "Greyscale Image"=w195, "Display"=w198, "slices"="slices", "dbg index"="dbg index") -> ("Greyscale Image 2"=w194:T16, "Detections"=w203:T18[], "gray"=→"gray":dbl, "2D Picture 2"=→"2D Picture 2":picture, "detect"=→"detect":dbl)  [unwired: 5 in, 1 out]
      }
      frame True {
      }
    }
    n67 = Tick Count (ms)() -> (millisecond timer value=w192:u32)
    n68 = feedback #2(w192) -> (w193:u32)
    n69 = feedback-in #2(w192) -> ()
    n70 = Subtract(x=w192, y=w193) -> (x-y=w175:u32)
    n71 = call <vilib>:"Butterworth Filter PtByPt.vi"("order"=5, "x"=w175) -> ("Filtered x"=→"Filtered x":dbl)  [unwired: 7 in, 1 out]
    n72 = call <vilib>:"Median Filter PtByPt.vi"("rank"=5, "x"=w175) -> ("Filtered x"=→"median of 5":dbl)  [unwired: 2 in, 1 out]
    n73 = Divide(x=w175, y=1000) -> (x/y=→"loop time (s)" →"Waveform Chart":dbl)
    n74 = call "Compute Tag Angles.vi"("Angle Mode"=w187, "Split Image Info"=w188, "IMU offset"="IMU offset", "tag info"=w189, "Detections"=w129) -> ("Vectors"=w159:cluster{cluster{"X":dbl, "Y":dbl}[]}[], "updated tags"=w137:T21)  [unwired: 5 in]
    "Tags" <- w137
    n75 = for {
      tunnel: w137 -> [w217] mode=indexing
      tunnel: [w214] -> w146 mode=indexing
      n76 = Unbundle By Name(w217) -> ("tag info.tag ID"=w215:i32, "Ange + Field Pos.angle"=w216:dbl)
      n77 = Bundle("tag ID"=w215, "angle"=w216) -> (w214:cluster{"tag ID":i32, "angle":dbl})  [unwired: 1 in]
    }
    "Tag & Angle" <- w146
    n78 = call "Build Combos.vi"("updated tags"=w137) -> ("Array"=w149:T22)  [unwired: 10 in]
    n79 = Unbundle("Circle Config") -> ("Sorting Mode"=w140:enum16{"Furthest Away", "Largest Radius"}, "How Many Circles?"=w142:dbl)
    n80 = case shown="\"Largest Radius\"" w140 {
      tunnel: w149 -> [w211 w213]
      tunnel: [w211 w212] -> w148
      frame "Furthest Away", Default {
      }
      frame "Largest Radius" {
        n81 = call "Sort Circles.vi"("Array 2"=w213) -> ("sorted array"=w212:T23)  [unwired: 10 in]
      }
    }
    n82 = for {
      tunnel: [w223] -> w147 mode=indexing
      tunnel: w148 -> [w222] mode=indexing
      n83 = Unbundle By Name(w222) -> ("Tag 1.tag info.tag ID"=w225:i32, "Tag 2.tag info.tag ID"=w224:i32, "Tag 1.Angle + Field Pos.angle"=w221:dbl, "Tag 2.Angle + Field Pos.angle"=w220:dbl)
      n84 = Subtract(x=w221, y=w220) -> (x-y=w219:dbl)
      n85 = Absolute Value(x=w219) -> (abs(x)=w218:dbl)
      n86 = Bundle("tag ID"=w225, "tag ID"=w224, w218) -> (w223:cluster{"tag ID":i32, "tag ID":i32, dbl})  [unwired: 1 in]
    }
    "Array 2" <- w147
    n87 = for {
      N: w142 -> [_]
      tunnel: w148 -> [w253] mode=indexing
      tunnel: [w244] -> w152 mode=indexing
      tunnel: [w246] -> w141 mode=indexing
      tunnel: [w245] -> w138 mode=indexing
      tunnel: [w244] -> w139 mode=indexing
      n88 = Unbundle(w253) -> ("Tag 1"=w252:T24, "Tag 2"=w251:T24)
      n89 = Unbundle(w252) -> ("Angle + Field Pos"=w247:T25)  [unwired: 1 out]
      n90 = Unbundle(w251) -> ("Angle + Field Pos"=w250:T25)  [unwired: 1 out]
      n91 = Bundle("Angle + Field Pos"=w247, "Angle + Field Pos"=w250) -> (w249:T26)  [unwired: 1 in]
      n92 = call "Chord to Center.vi"("Tag points"=w249) -> ("output circle info"=w244:T27)  [unwired: 7 in, 3 out]
      n93 = call "Create Circle Plot.vi"("Circle Descr"=w244) -> ("Points"=w248:cluster{dbl, dbl}[])  [unwired: 10 in]
      n94 = Bundle("Points"=w248) -> (w245:cluster{"Points":cluster{dbl, dbl}[]})  [unwired: 1 in]
      n95 = Bundle("output circle info"=w244, w245) -> (w246:T28)  [unwired: 1 in]
    }
    n96 = case shown="\"Furthest Away\"" w140 {
      tunnel: [w208 w210] -> w145
      tunnel: [w207 w209] -> w144
      tunnel: w141 -> [w206 _]
      tunnel: w139 -> [_ w210]
      tunnel: w138 -> [_ w209]
      frame "Furthest Away" {
        n97 = call "Sort Circle Center.vi"("Array 3"=w206) -> ("Circle Plots"=w207:cluster{"Points":cluster{dbl, dbl}[]}[], "Circle Combos"=w208:T29)  [unwired: 9 in]
      }
      frame Default {
      }
    }
    n98 = for {
      N -> [w227]
      tunnel: w145 -> [w232] mode=indexing
      tunnel: w145 -> [w231]
      tunnel: [w226] -> w150 mode=concatenating
      i -> [w229]
      # "build combos"
      n99 = Compound Arithmetic op=ADD(w227, invert 1 ("value"), invert w229) -> (w230:i32)
      n100 = for {
        N: w230 -> [_]
        tunnel: w232 -> [w238]
        tunnel: w231 -> [w243]
        tunnel: w229 -> [w241]
        tunnel: [w234] -> w226 mode=indexing
        i -> [w240]
        n101 = Compound Arithmetic op=ADD(w241, w240, 1 ("value")) -> (w242:i32)
        n102 = Index Array(array=w243, index=w242) -> (element=w237:T27)
        n103 = call "Intersect Circles.vi"("Circle 2"=w237, "Circle 1"=w238) -> ("Point 2"=w235:cluster{dbl, dbl}, "Point 1"=w236:cluster{dbl, dbl})  [unwired: 8 in]
        n104 = Build Array(w236, w235) -> (w233:cluster{dbl, dbl}[])
        n105 = Bundle(w233) -> (w234:cluster{cluster{dbl, dbl}[]})  [unwired: 1 in]
      }
    }
    n106 = call "Get Robot Pose Coordinates.vi"("Intersection Points"=w150, "Circle Points"=w152, "April Tag Info"=w189, "IMU value"="IMU value") -> ("Robot Pose"=w179:cluster{dbl, dbl})  [unwired: 6 in]
    n107 = Bundle By Name(cluster=w162, "Name"="Robot Pose", "Position"=w179, "Color"=u32 16711680, "Point Style"=5, "Name Visible"=TRUE) -> (w136:T7)
    n108 = call "Get Cursors.vi"("tag info not from game manual"=w189, "Detections"=w129, "Cluster"=w162) -> ("Array"=w132:T30)  [unwired: 8 in]
    n109 = Select(t=w150, s="Chords", f=w190) -> (s? t:f=w155:cluster{cluster{"X":dbl, "Y":dbl}[]}[])
    n110 = Select(t=w144, s="Circles", f=w190) -> (s? t:f=w156:cluster{"Points":cluster{"X":dbl, "Y":dbl}[]}[])
    n111 = Select(t=w159, s="Lines", f=w190) -> (s? t:f=w158:cluster{cluster{"X":dbl, "Y":dbl}[]}[])
    n112 = Build Array (concatenate)(w132, w136) -> (w135:T30)
    n113 = Build Array (concatenate)(w158, w155, w156) -> (→"Field":cluster{"Points":cluster{"X":dbl, "Y":dbl}[]}[])
    n114 = property on="Field" class="XYGraph (strict)"("CrsrList"=w135) -> ()  [unwired: 2 in, 2 out]
    n115 = disable-structure shown="Enabled" {
      disable-tunnel: w182 -> [w281 _]
      disable-tunnel: w181 -> [w280 _]
      disable-tunnel: w180 -> [w279 _]
      disable-tunnel: w129 -> [w278 _]
      disable-tunnel: w179 -> [w277 _]
      frame Enabled {
        n116 = local read "sorted array"() -> (w274:T1)
        n117 = Bundle("Detections"=w278, "Robot Pose"=w277, "sorted array"=w274) -> (w273:T31)  [unwired: 1 in]
        n118 = Flatten To String(anything=w273) -> (data string=w276:string)  [unwired: 3 in, 2 out]
        n119 = UDP Write(address=w280, port or service name=w281, connection ID=w279, data in=w276, 9:1 ("timeout ms (25000)")) -> (error out=→"error out 2":errorcluster)  [unwired: 1 in, 1 out]
      }
      frame Disabled {
      }
    }
    n120 = call <vilib>:"ARGB Image to Greyscale Image.vi"("Greyscale Image Destination in"=w116, "ARGB Image Source in"=w122) -> ("Greyscale Image Destination"=w121:T16)  [unwired: 8 in, 1 out]
    "Timed Out?" <- w173
    "Acquire" <- w164
  }
  n121 = disable-structure shown="Disabled" {
    disable-tunnel: w30 -> [w283 _]
    frame Disabled {
      n122 = call <vilib>:"Stop.vi"("Stream in"=w283) -> ("Stream"=w284:refnum<class "Stream.lvclass">)  [unwired: 9 in, 1 out]
      n123 = call <vilib>:"Destroy.vi"("Stream in"=w284) -> ()  [unwired: 10 in, 1 out]
    }
    frame Enabled {
    }
  }
